vi "SelectRobotConfig.vi"(1 "RobotID":T19) -> (0 "RobotConfig":T1={"Motors"={"RightDrivePrimary"={"CAN Address"=0, "Invert"=FALSE, "InvertSensor"=FALSE, "Unit Conversion Factor"=0.0, "Brake Mode"=enum."Override to Brake", "Reverse Limt Switch Mode"=enum."Disabled", "Forward Limt Swith Mode"=enum."Disabled", "PWM Channel"=enum."Invalid", "Motor Controller Type"=enum."Talon SRX", "Peak Current (A)"=0, "Continuous Current (A)"=0, "Peak Duration (ms)"=0, "Current Limit Enable"=FALSE}, "RightDriveSecondary"={"CAN Address"=0, "Invert"=FALSE, "InvertSensor"=FALSE, "Unit Conversion Factor"=0.0, "Brake Mode"=enum."Override to Brake", "Reverse Limt Switch Mode"=enum."Disabled", "Forward Limt Swith Mode"=enum."Disabled", "PWM Channel"=enum."Invalid", "Motor Controller Type"=enum."Talon SRX", "Peak Current (A)"=0, "Continuous Current (A)"=0, "Peak Duration (ms)"=0, "Current Limit Enable"=FALSE}, "LeftDrivePrimary"={"CAN Address"=0, "Invert"=FALSE, "InvertSensor"=FALSE, "Unit Conversion Factor"=0.0, "Brake Mode"=enum."Override to Brake", "Reverse Limt Switch Mode"=enum."Disabled", "Forward Limt Swith Mode"=enum."Disabled", "PWM Channel"=enum."Invalid", "Motor Controller Type"=enum."Talon SRX", "Peak Current (A)"=0, "Continuous Current (A)"=0, "Peak Duration (ms)"=0, "Current Limit Enable"=FALSE}, "LeftDriveSecondary"={"CAN Address"=0, "Invert"=FALSE, "InvertSensor"=FALSE, "Unit Conversion Factor"=0.0, "Brake Mode"=enum."Override to Brake", "Reverse Limt Switch Mode"=enum."Disabled", "Forward Limt Swith Mode"=enum."Disabled", "PWM Channel"=enum."Invalid", "Motor Controller Type"=enum."Talon SRX", "Peak Current (A)"=0, "Continuous Current (A)"=0, "Peak Duration (ms)"=0, "Current Limit Enable"=FALSE}, "RightShooter"={"CAN Address"=0, "Invert"=FALSE, "InvertSensor"=FALSE, "Unit Conversion Factor"=0.0, "Brake Mode"=enum."Override to Brake", "Reverse Limt Switch Mode"=enum."Disabled", "Forward Limt Swith Mode"=enum."Disabled", "PWM Channel"=enum."Invalid", "Motor Controller Type"=enum."Talon SRX", "Peak Current (A)"=0, "Continuous Current (A)"=0, "Peak Duration (ms)"=0, "Current Limit Enable"=FALSE}, "LeftShooter"={"CAN Address"=0, "Invert"=FALSE, "InvertSensor"=FALSE, "Unit Conversion Factor"=0.0, "Brake Mode"=enum."Override to Brake", "Reverse Limt Switch Mode"=enum."Disabled", "Forward Limt Swith Mode"=enum."Disabled", "PWM Channel"=enum."Invalid", "Motor Controller Type"=enum."Talon SRX", "Peak Current (A)"=0, "Continuous Current (A)"=0, "Peak Duration (ms)"=0, "Current Limit Enable"=FALSE}, "ShooterRotate"={"CAN Address"=0, "Invert"=FALSE, "InvertSensor"=FALSE, "Unit Conversion Factor"=0.0, "Brake Mode"=enum."Override to Brake", "Reverse Limt Switch Mode"=enum."Disabled", "Forward Limt Swith Mode"=enum."Disabled", "PWM Channel"=enum."Invalid", "Motor Controller Type"=enum."Talon SRX", "Peak Current (A)"=0, "Continuous Current (A)"=0, "Peak Duration (ms)"=0, "Current Limit Enable"=FALSE}, "ShooterHood"={"CAN Address"=0, "Invert"=FALSE, "InvertSensor"=FALSE, "Unit Conversion Factor"=0.0, "Brake Mode"=enum."Override to Brake", "Reverse Limt Switch Mode"=enum."Disabled", "Forward Limt Swith Mode"=enum."Disabled", "PWM Channel"=enum."Invalid", "Motor Controller Type"=enum."Talon SRX", "Peak Current (A)"=0, "Continuous Current (A)"=0, "Peak Duration (ms)"=0, "Current Limit Enable"=FALSE}, "HopperWheel"={"CAN Address"=0, "Invert"=FALSE, "InvertSensor"=FALSE, "Unit Conversion Factor"=0.0, "Brake Mode"=enum."Override to Brake", "Reverse Limt Switch Mode"=enum."Disabled", "Forward Limt Swith Mode"=enum."Disabled", "PWM Channel"=enum."Invalid", "Motor Controller Type"=enum."Talon SRX", "Peak Current (A)"=0, "Continuous Current (A)"=0, "Peak Duration (ms)"=0, "Current Limit Enable"=FALSE}, "Elevator"={"CAN Address"=0, "Invert"=FALSE, "InvertSensor"=FALSE, "Unit Conversion Factor"=0.0, "Brake Mode"=enum."Override to Brake", "Reverse Limt Switch Mode"=enum."Disabled", "Forward Limt Swith Mode"=enum."Disabled", "PWM Channel"=enum."Invalid", "Motor Controller Type"=enum."Talon SRX", "Peak Current (A)"=0, "Continuous Current (A)"=0, "Peak Duration (ms)"=0, "Current Limit Enable"=FALSE}, "ClimberLeft"={"CAN Address"=0, "Invert"=FALSE, "InvertSensor"=FALSE, "Unit Conversion Factor"=0.0, "Brake Mode"=enum."Override to Brake", "Reverse Limt Switch Mode"=enum."Disabled", "Forward Limt Swith Mode"=enum."Disabled", "PWM Channel"=enum."Invalid", "Motor Controller Type"=enum."Talon SRX", "Peak Current (A)"=0, "Continuous Current (A)"=0, "Peak Duration (ms)"=0, "Current Limit Enable"=FALSE}, "ClimberRight"={"CAN Address"=0, "Invert"=FALSE, "InvertSensor"=FALSE, "Unit Conversion Factor"=0.0, "Brake Mode"=enum."Override to Brake", "Reverse Limt Switch Mode"=enum."Disabled", "Forward Limt Swith Mode"=enum."Disabled", "PWM Channel"=enum."Invalid", "Motor Controller Type"=enum."Talon SRX", "Peak Current (A)"=0, "Continuous Current (A)"=0, "Peak Duration (ms)"=0, "Current Limit Enable"=FALSE}, "Intake"={"CAN Address"=0, "Invert"=FALSE, "InvertSensor"=FALSE, "Unit Conversion Factor"=0.0, "Brake Mode"=enum."Override to Brake", "Reverse Limt Switch Mode"=enum."Disabled", "Forward Limt Swith Mode"=enum."Disabled", "PWM Channel"=enum."Invalid", "Motor Controller Type"=enum."Talon SRX", "Peak Current (A)"=0, "Continuous Current (A)"=0, "Peak Duration (ms)"=0, "Current Limit Enable"=FALSE}, "ControlPanel"={"CAN Address"=0, "Invert"=FALSE, "InvertSensor"=FALSE, "Unit Conversion Factor"=0.0, "Brake Mode"=enum."Override to Brake", "Reverse Limt Switch Mode"=enum."Disabled", "Forward Limt Swith Mode"=enum."Disabled", "PWM Channel"=enum."Invalid", "Motor Controller Type"=enum."Talon SRX", "Peak Current (A)"=0, "Continuous Current (A)"=0, "Peak Duration (ms)"=0, "Current Limit Enable"=FALSE}}, "PID"={"Shooter"={"P"=0.0, "I"=0.0, "D"=0.0, "F"=0.0, "IZone"=0.0}, "Turret"={"P"=0.0, "I"=0.0, "D"=0.0, "F"=0.0, "IZone"=0.0}, "Elevator"={"P"=0.0, "I"=0.0, "D"=0.0, "F"=0.0, "IZone"=0.0}, "ControlPanel"={"P"=0.0, "I"=0.0, "D"=0.0, "F"=0.0, "IZone"=0.0}, "Hood"={"P"=0.0, "I"=0.0, "D"=0.0, "F"=0.0, "IZone"=0.0}}, "MotionMagic"={"Turret"={"CruiseVelocity"=0, "Acceleration"=0}, "Elevator"={"CruiseVelocity"=0, "Acceleration"=0}, "ControlPanel"={"CruiseVelocity"=0, "Acceleration"=0}}, "Sensors"={"IMU"={"Yaw Axis"=enum."Z", "SPI Bus"=enum."SPI MXP", "AHRS Algorithm"=enum."Complementary", "Calibration Time (s)"=3.0, "Calibrate On Open"=TRUE}, "ElevatorBottom"={"ID"=0, "RangingMode"=enum."Short", "sampleTime(ms)"=24.0}, "ElevatorTop"={"ID"=0, "RangingMode"=enum."Short", "sampleTime(ms)"=24.0}, "ControlPanelColorSensor"={"alsIntegrationTime(ms)"=10.0, "alsGain"=40, "I2C Bus"=enum."I2C On-Board", "numProximityPulses"=5, "proximityGain"=1, "proximityLEDCurrent(mA)"=50, "proximityPulseLength(ms)"=0.01, "proximitySampleTime(ms)"=10.0}}, "Solenoids"={"Intake"={"SolenoidChannel"=enum."Solenoid 0", "Invert"=FALSE}, "ClimberRachet"={"SolenoidChannel"=enum."Solenoid 0", "Invert"=FALSE}}, "EnableCompressor"=FALSE, "RobotDimensions"={"Wheelbase(in)"=0.0, "Length(in)"=0.0}, "CameraMounting"={"LensHeight(in)"=0.0, "RotationRadius(in)"=0.0, "Pitch(deg)"=0.0}, "SensorCalibrations"={"TopToFMinBallDistance(in)"=0.0, "BottomToFMinBallDistance(in)"=0.0}, "Homing"={"Hood Homing Position (deg)"=0.0, "Turret Homing Position (deg)"=0.0}, "MotionLimits"={"Hood"={"Min (deg)"=0.0, "Max (deg)"=0.0}, "Turret"={"Min (deg)"=0.0, "Max (deg)"=0.0}}} {"Sensors"."ElevatorTop"."sampleTime(ms)" min=24.0 max=1000.0 step=1.0; "Sensors"."ElevatorBottom"."sampleTime(ms)" min=24.0 max=1000.0 step=1.0})   [LabVIEW 2019]
uses:
  TypeDefs/RobotID.ctl
  TypeDefs/ConfigComponents/Config_Robot.ctl
  ArgosLib/Config/ConfigComponents/TypeDefs/Config_Motor.ctl
  <vilib>/Rock Robotics/WPI/ThirdParty/Phoenix-LabVIEW/Motor Controller/Controls/CTRE_Phoenix_MotorControl_NeutralMode.ctl
  <vilib>/Rock Robotics/WPI/ThirdParty/Phoenix-LabVIEW/Motor Controller/Controls/CTRE_Phoenix_MotorControl_LimitSwitchNormal.ctl
  <vilib>/Rock Robotics/SystemInterfaces/DIO/FPGA_DIOPWMChannel.ctl
  ArgosLib/Config/ConfigComponents/TypeDefs/Config_MotorCtrlType.ctl
  ArgosLib/Config/ConfigComponents/TypeDefs/Config_PIDParams.ctl
  ArgosLib/Config/ConfigComponents/TypeDefs/Config_MotionMagicParams.ctl
  ArgosLib/Config/ConfigComponents/TypeDefs/Config_IMU.ctl
  <vilib>/Rock Robotics/SystemInterfaces/spilib/spi_bus.ctl
  ArgosLib/Config/ConfigComponents/TypeDefs/Config_PwFToF.ctl
  <vilib>/Playing With Fusion Inc/Playing With Fusion Lib for FRC/PWF_ToF_LabVIEW/Public/TypeDefs/PwF_ToF_RangingMode.ctl
  ArgosLib/Config/ConfigComponents/TypeDefs/Config_PwF_TMD37003.ctl
  <vilib>/Rock Robotics/SystemInterfaces/i2clib/i2c_bus.ctl
  ArgosLib/Config/ConfigComponents/TypeDefs/Config_SingleSolenoid.ctl
  <vilib>/Rock Robotics/WPI/Solenoid/WPI_SolenoidChannel.ctl
  TypeDefs/ConfigComponents/Config_RobotDimensions.ctl
  TypeDefs/ConfigComponents/Config_CameraMounting.ctl
  ArgosLib/ArgosLib.lvlib
  <vilib>/Playing With Fusion Inc/Playing With Fusion Lib for FRC/PWF_ToF_LabVIEW/PwF_ToF.lvlib
panel:
  in  "Competition":T1={"Motors"={"RightDrivePrimary"={"CAN Address"=1, "Invert"=TRUE, "InvertSensor"=FALSE, "Unit Conversion Factor"=0.4342, "Brake Mode"=enum."Override to Brake", "Reverse Limt Switch Mode"=enum."Disabled", "Forward Limt Swith Mode"=enum."Disabled", "PWM Channel"=enum."Invalid", "Motor Controller Type"=enum."Venom", "Peak Current (A)"=0, "Continuous Current (A)"=0, "Peak Duration (ms)"=0, "Current Limit Enable"=FALSE}, "RightDriveSecondary"={"CAN Address"=2, "Invert"=TRUE, "InvertSensor"=FALSE, "Unit Conversion Factor"=0.4342, "Brake Mode"=enum."Override to Brake", "Reverse Limt Switch Mode"=enum."Disabled", "Forward Limt Swith Mode"=enum."Disabled", "PWM Channel"=enum."Invalid", "Motor Controller Type"=enum."Venom", "Peak Current (A)"=0, "Continuous Current (A)"=0, "Peak Duration (ms)"=0, "Current Limit Enable"=FALSE}, "LeftDrivePrimary"={"CAN Address"=3, "Invert"=FALSE, "InvertSensor"=FALSE, "Unit Conversion Factor"=0.4342, "Brake Mode"=enum."Override to Brake", "Reverse Limt Switch Mode"=enum."Disabled", "Forward Limt Swith Mode"=enum."Disabled", "PWM Channel"=enum."Invalid", "Motor Controller Type"=enum."Venom", "Peak Current (A)"=0, "Continuous Current (A)"=0, "Peak Duration (ms)"=0, "Current Limit Enable"=FALSE}, "LeftDriveSecondary"={"CAN Address"=4, "Invert"=FALSE, "InvertSensor"=FALSE, "Unit Conversion Factor"=0.4342, "Brake Mode"=enum."Override to Brake", "Reverse Limt Switch Mode"=enum."Disabled", "Forward Limt Swith Mode"=enum."Disabled", "PWM Channel"=enum."Invalid", "Motor Controller Type"=enum."Venom", "Peak Current (A)"=0, "Continuous Current (A)"=0, "Peak Duration (ms)"=0, "Current Limit Enable"=FALSE}, "RightShooter"={"CAN Address"=5, "Invert"=FALSE, "InvertSensor"=FALSE, "Unit Conversion Factor"=1228.8, "Brake Mode"=enum."Override to Coast", "Reverse Limt Switch Mode"=enum."Disabled", "Forward Limt Swith Mode"=enum."Disabled", "PWM Channel"=enum."Invalid", "Motor Controller Type"=enum."Falcon FX", "Peak Current (A)"=0, "Continuous Current (A)"=0, "Peak Duration (ms)"=0, "Current Limit Enable"=FALSE}, "LeftShooter"={"CAN Address"=6, "Invert"=TRUE, "InvertSensor"=FALSE, "Unit Conversion Factor"=1228.8, "Brake Mode"=enum."Override to Coast", "Reverse Limt Switch Mode"=enum."Disabled", "Forward Limt Swith Mode"=enum."Disabled", "PWM Channel"=enum."Invalid", "Motor Controller Type"=enum."Falcon FX", "Peak Current (A)"=0, "Continuous Current (A)"=0, "Peak Duration (ms)"=0, "Current Limit Enable"=FALSE}, "ShooterRotate"={"CAN Address"=7, "Invert"=TRUE, "InvertSensor"=TRUE, "Unit Conversion Factor"=11.3777, "Brake Mode"=enum."Override to Brake", "Reverse Limt Switch Mode"=enum."Disabled", "Forward Limt Swith Mode"=enum."Disabled", "PWM Channel"=enum."Invalid", "Motor Controller Type"=enum."Talon SRX", "Peak Current (A)"=0, "Continuous Current (A)"=0, "Peak Duration (ms)"=0, "Current Limit Enable"=FALSE}, "ShooterHood"={"CAN Address"=8, "Invert"=FALSE, "InvertSensor"=FALSE, "Unit Conversion Factor"=153.949, "Brake Mode"=enum."Override to Brake", "Reverse Limt Switch Mode"=enum."Disabled", "Forward Limt Swith Mode"=enum."Disabled", "PWM Channel"=enum."Invalid", "Motor Controller Type"=enum."Talon SRX", "Peak Current (A)"=0, "Continuous Current (A)"=0, "Peak Duration (ms)"=0, "Current Limit Enable"=FALSE}, "HopperWheel"={"CAN Address"=9, "Invert"=FALSE, "InvertSensor"=FALSE, "Unit Conversion Factor"=0.0, "Brake Mode"=enum."Override to Brake", "Reverse Limt Switch Mode"=enum."Disabled", "Forward Limt Swith Mode"=enum."Disabled", "PWM Channel"=enum."Invalid", "Motor Controller Type"=enum."Talon SRX", "Peak Current (A)"=0, "Continuous Current (A)"=0, "Peak Duration (ms)"=0, "Current Limit Enable"=FALSE}, "Elevator"={"CAN Address"=10, "Invert"=FALSE, "InvertSensor"=FALSE, "Unit Conversion Factor"=0.0, "Brake Mode"=enum."Override to Brake", "Reverse Limt Switch Mode"=enum."Disabled", "Forward Limt Swith Mode"=enum."Disabled", "PWM Channel"=enum."Invalid", "Motor Controller Type"=enum."Talon SRX", "Peak Current (A)"=0, "Continuous Current (A)"=0, "Peak Duration (ms)"=0, "Current Limit Enable"=FALSE}, "ClimberLeft"={"CAN Address"=11, "Invert"=TRUE, "InvertSensor"=FALSE, "Unit Conversion Factor"=0.0, "Brake Mode"=enum."Override to Brake", "Reverse Limt Switch Mode"=enum."Disabled", "Forward Limt Swith Mode"=enum."Disabled", "PWM Channel"=enum."Invalid", "Motor Controller Type"=enum."Talon SRX", "Peak Current (A)"=0, "Continuous Current (A)"=0, "Peak Duration (ms)"=0, "Current Limit Enable"=FALSE}, "ClimberRight"={"CAN Address"=12, "Invert"=FALSE, "InvertSensor"=FALSE, "Unit Conversion Factor"=0.0, "Brake Mode"=enum."Override to Brake", "Reverse Limt Switch Mode"=enum."Disabled", "Forward Limt Swith Mode"=enum."Disabled", "PWM Channel"=enum."Invalid", "Motor Controller Type"=enum."Talon SRX", "Peak Current (A)"=0, "Continuous Current (A)"=0, "Peak Duration (ms)"=0, "Current Limit Enable"=FALSE}, "Intake"={"CAN Address"=13, "Invert"=TRUE, "InvertSensor"=FALSE, "Unit Conversion Factor"=0.0, "Brake Mode"=enum."Override to Brake", "Reverse Limt Switch Mode"=enum."Disabled", "Forward Limt Swith Mode"=enum."Disabled", "PWM Channel"=enum."Invalid", "Motor Controller Type"=enum."Talon SRX", "Peak Current (A)"=0, "Continuous Current (A)"=0, "Peak Duration (ms)"=0, "Current Limit Enable"=FALSE}, "ControlPanel"={"CAN Address"=14, "Invert"=FALSE, "InvertSensor"=FALSE, "Unit Conversion Factor"=0.0, "Brake Mode"=enum."Override to Brake", "Reverse Limt Switch Mode"=enum."Disabled", "Forward Limt Swith Mode"=enum."Disabled", "PWM Channel"=enum."Invalid", "Motor Controller Type"=enum."Talon SRX", "Peak Current (A)"=0, "Continuous Current (A)"=0, "Peak Duration (ms)"=0, "Current Limit Enable"=FALSE}}, "PID"={"Shooter"={"P"=1.0, "I"=0.001, "D"=0.0, "F"=0.055, "IZone"=200.0}, "Turret"={"P"=6.0, "I"=0.1, "D"=0.0, "F"=0.0, "IZone"=500.0}, "Elevator"={"P"=0.0, "I"=0.0, "D"=0.0, "F"=0.0, "IZone"=0.0}, "ControlPanel"={"P"=0.0, "I"=0.0, "D"=0.0, "F"=0.0, "IZone"=0.0}, "Hood"={"P"=0.5, "I"=0.0007, "D"=0.0, "F"=0.0, "IZone"=200.0}}, "MotionMagic"={"Turret"={"CruiseVelocity"=0, "Acceleration"=0}, "Elevator"={"CruiseVelocity"=0, "Acceleration"=0}, "ControlPanel"={"CruiseVelocity"=0, "Acceleration"=0}}, "Sensors"={"IMU"={"Yaw Axis"=enum."Z", "SPI Bus"=enum."SPI MXP", "AHRS Algorithm"=enum."Complementary", "Calibration Time (s)"=3.0, "Calibrate On Open"=TRUE}, "ElevatorBottom"={"ID"=1, "RangingMode"=enum."Short", "sampleTime(ms)"=24.0}, "ElevatorTop"={"ID"=2, "RangingMode"=enum."Short", "sampleTime(ms)"=24.0}, "ControlPanelColorSensor"={"alsIntegrationTime(ms)"=10.0, "alsGain"=40, "I2C Bus"=enum."I2C On-Board", "numProximityPulses"=5, "proximityGain"=1, "proximityLEDCurrent(mA)"=50, "proximityPulseLength(ms)"=0.01, "proximitySampleTime(ms)"=10.0}}, "Solenoids"={"Intake"={"SolenoidChannel"=enum."Solenoid 0", "Invert"=FALSE}, "ClimberRachet"={"SolenoidChannel"=enum."Solenoid 1", "Invert"=FALSE}}, "EnableCompressor"=TRUE, "RobotDimensions"={"Wheelbase(in)"=0.0, "Length(in)"=0.0}, "CameraMounting"={"LensHeight(in)"=37.75, "RotationRadius(in)"=7.0, "Pitch(deg)"=24.5}, "SensorCalibrations"={"TopToFMinBallDistance(in)"=1.0, "BottomToFMinBallDistance(in)"=0.0}, "Homing"={"Hood Homing Position (deg)"=45.0, "Turret Homing Position (deg)"=0.0}, "MotionLimits"={"Hood"={"Min (deg)"=47.0, "Max (deg)"=72.0}, "Turret"={"Min (deg)"=-108.0, "Max (deg)"=108.0}}} {"Sensors"."ElevatorTop"."sampleTime(ms)" min=24.0 max=1000.0 step=1.0; "Sensors"."ElevatorBottom"."sampleTime(ms)" min=24.0 max=1000.0 step=1.0}
  in  "Practice":T1={"Motors"={"RightDrivePrimary"={"CAN Address"=1, "Invert"=TRUE, "InvertSensor"=FALSE, "Unit Conversion Factor"=0.4342, "Brake Mode"=enum."Override to Brake", "Reverse Limt Switch Mode"=enum."Disabled", "Forward Limt Swith Mode"=enum."Disabled", "PWM Channel"=enum."Invalid", "Motor Controller Type"=enum."Venom", "Peak Current (A)"=0, "Continuous Current (A)"=0, "Peak Duration (ms)"=0, "Current Limit Enable"=FALSE}, "RightDriveSecondary"={"CAN Address"=2, "Invert"=TRUE, "InvertSensor"=FALSE, "Unit Conversion Factor"=0.4342, "Brake Mode"=enum."Override to Brake", "Reverse Limt Switch Mode"=enum."Disabled", "Forward Limt Swith Mode"=enum."Disabled", "PWM Channel"=enum."Invalid", "Motor Controller Type"=enum."Venom", "Peak Current (A)"=0, "Continuous Current (A)"=0, "Peak Duration (ms)"=0, "Current Limit Enable"=FALSE}, "LeftDrivePrimary"={"CAN Address"=3, "Invert"=FALSE, "InvertSensor"=FALSE, "Unit Conversion Factor"=0.4342, "Brake Mode"=enum."Override to Brake", "Reverse Limt Switch Mode"=enum."Disabled", "Forward Limt Swith Mode"=enum."Disabled", "PWM Channel"=enum."Invalid", "Motor Controller Type"=enum."Venom", "Peak Current (A)"=0, "Continuous Current (A)"=0, "Peak Duration (ms)"=0, "Current Limit Enable"=FALSE}, "LeftDriveSecondary"={"CAN Address"=4, "Invert"=FALSE, "InvertSensor"=FALSE, "Unit Conversion Factor"=0.4342, "Brake Mode"=enum."Override to Brake", "Reverse Limt Switch Mode"=enum."Disabled", "Forward Limt Swith Mode"=enum."Disabled", "PWM Channel"=enum."Invalid", "Motor Controller Type"=enum."Venom", "Peak Current (A)"=0, "Continuous Current (A)"=0, "Peak Duration (ms)"=0, "Current Limit Enable"=FALSE}, "RightShooter"={"CAN Address"=5, "Invert"=TRUE, "InvertSensor"=FALSE, "Unit Conversion Factor"=1228.8, "Brake Mode"=enum."Override to Coast", "Reverse Limt Switch Mode"=enum."Disabled", "Forward Limt Swith Mode"=enum."Disabled", "PWM Channel"=enum."Invalid", "Motor Controller Type"=enum."Falcon FX", "Peak Current (A)"=0, "Continuous Current (A)"=0, "Peak Duration (ms)"=0, "Current Limit Enable"=FALSE}, "LeftShooter"={"CAN Address"=6, "Invert"=FALSE, "InvertSensor"=FALSE, "Unit Conversion Factor"=1228.8, "Brake Mode"=enum."Override to Coast", "Reverse Limt Switch Mode"=enum."Disabled", "Forward Limt Swith Mode"=enum."Disabled", "PWM Channel"=enum."Invalid", "Motor Controller Type"=enum."Falcon FX", "Peak Current (A)"=0, "Continuous Current (A)"=0, "Peak Duration (ms)"=0, "Current Limit Enable"=FALSE}, "ShooterRotate"={"CAN Address"=7, "Invert"=TRUE, "InvertSensor"=FALSE, "Unit Conversion Factor"=11.3777, "Brake Mode"=enum."Override to Brake", "Reverse Limt Switch Mode"=enum."Disabled", "Forward Limt Swith Mode"=enum."Disabled", "PWM Channel"=enum."Invalid", "Motor Controller Type"=enum."Talon SRX", "Peak Current (A)"=0, "Continuous Current (A)"=0, "Peak Duration (ms)"=0, "Current Limit Enable"=FALSE}, "ShooterHood"={"CAN Address"=8, "Invert"=FALSE, "InvertSensor"=FALSE, "Unit Conversion Factor"=442.112, "Brake Mode"=enum."Override to Brake", "Reverse Limt Switch Mode"=enum."Disabled", "Forward Limt Swith Mode"=enum."Disabled", "PWM Channel"=enum."Invalid", "Motor Controller Type"=enum."Talon SRX", "Peak Current (A)"=0, "Continuous Current (A)"=0, "Peak Duration (ms)"=0, "Current Limit Enable"=FALSE}, "HopperWheel"={"CAN Address"=9, "Invert"=FALSE, "InvertSensor"=FALSE, "Unit Conversion Factor"=0.0, "Brake Mode"=enum."Override to Brake", "Reverse Limt Switch Mode"=enum."Disabled", "Forward Limt Swith Mode"=enum."Disabled", "PWM Channel"=enum."Invalid", "Motor Controller Type"=enum."Talon SRX", "Peak Current (A)"=0, "Continuous Current (A)"=0, "Peak Duration (ms)"=0, "Current Limit Enable"=FALSE}, "Elevator"={"CAN Address"=10, "Invert"=FALSE, "InvertSensor"=FALSE, "Unit Conversion Factor"=0.0, "Brake Mode"=enum."Override to Brake", "Reverse Limt Switch Mode"=enum."Disabled", "Forward Limt Swith Mode"=enum."Disabled", "PWM Channel"=enum."Invalid", "Motor Controller Type"=enum."Talon SRX", "Peak Current (A)"=0, "Continuous Current (A)"=0, "Peak Duration (ms)"=0, "Current Limit Enable"=FALSE}, "ClimberLeft"={"CAN Address"=11, "Invert"=FALSE, "InvertSensor"=FALSE, "Unit Conversion Factor"=0.0, "Brake Mode"=enum."Override to Brake", "Reverse Limt Switch Mode"=enum."Disabled", "Forward Limt Swith Mode"=enum."Disabled", "PWM Channel"=enum."Invalid", "Motor Controller Type"=enum."Talon SRX", "Peak Current (A)"=0, "Continuous Current (A)"=0, "Peak Duration (ms)"=0, "Current Limit Enable"=FALSE}, "ClimberRight"={"CAN Address"=12, "Invert"=FALSE, "InvertSensor"=FALSE, "Unit Conversion Factor"=0.0, "Brake Mode"=enum."Override to Brake", "Reverse Limt Switch Mode"=enum."Disabled", "Forward Limt Swith Mode"=enum."Disabled", "PWM Channel"=enum."Invalid", "Motor Controller Type"=enum."Talon SRX", "Peak Current (A)"=0, "Continuous Current (A)"=0, "Peak Duration (ms)"=0, "Current Limit Enable"=FALSE}, "Intake"={"CAN Address"=13, "Invert"=TRUE, "InvertSensor"=FALSE, "Unit Conversion Factor"=0.0, "Brake Mode"=enum."Override to Brake", "Reverse Limt Switch Mode"=enum."Disabled", "Forward Limt Swith Mode"=enum."Disabled", "PWM Channel"=enum."Invalid", "Motor Controller Type"=enum."Talon SRX", "Peak Current (A)"=0, "Continuous Current (A)"=0, "Peak Duration (ms)"=0, "Current Limit Enable"=FALSE}, "ControlPanel"={"CAN Address"=14, "Invert"=FALSE, "InvertSensor"=FALSE, "Unit Conversion Factor"=0.0, "Brake Mode"=enum."Override to Brake", "Reverse Limt Switch Mode"=enum."Disabled", "Forward Limt Swith Mode"=enum."Disabled", "PWM Channel"=enum."Invalid", "Motor Controller Type"=enum."Talon SRX", "Peak Current (A)"=0, "Continuous Current (A)"=0, "Peak Duration (ms)"=0, "Current Limit Enable"=FALSE}}, "PID"={"Shooter"={"P"=0.0004, "I"=1e-06, "D"=0.0, "F"=0.0002, "IZone"=200.0}, "Turret"={"P"=6.0, "I"=0.007, "D"=0.0, "F"=0.0, "IZone"=500.0}, "Elevator"={"P"=0.0, "I"=0.0, "D"=0.0, "F"=0.0, "IZone"=0.0}, "ControlPanel"={"P"=0.0, "I"=0.0, "D"=0.0, "F"=0.0, "IZone"=0.0}, "Hood"={"P"=0.3, "I"=0.0001, "D"=0.0, "F"=0.0, "IZone"=1000.0}}, "MotionMagic"={"Turret"={"CruiseVelocity"=0, "Acceleration"=0}, "Elevator"={"CruiseVelocity"=0, "Acceleration"=0}, "ControlPanel"={"CruiseVelocity"=0, "Acceleration"=0}}, "Sensors"={"IMU"={"Yaw Axis"=enum."Z", "SPI Bus"=enum."SPI MXP", "AHRS Algorithm"=enum."Complementary", "Calibration Time (s)"=3.0, "Calibrate On Open"=TRUE}, "ElevatorBottom"={"ID"=1, "RangingMode"=enum."Short", "sampleTime(ms)"=24.0}, "ElevatorTop"={"ID"=2, "RangingMode"=enum."Short", "sampleTime(ms)"=24.0}, "ControlPanelColorSensor"={"alsIntegrationTime(ms)"=10.0, "alsGain"=40, "I2C Bus"=enum."I2C On-Board", "numProximityPulses"=5, "proximityGain"=1, "proximityLEDCurrent(mA)"=50, "proximityPulseLength(ms)"=0.01, "proximitySampleTime(ms)"=10.0}}, "Solenoids"={"Intake"={"SolenoidChannel"=enum."Solenoid 0", "Invert"=TRUE}, "ClimberRachet"={"SolenoidChannel"=enum."Solenoid 1", "Invert"=FALSE}}, "EnableCompressor"=FALSE, "RobotDimensions"={"Wheelbase(in)"=0.0, "Length(in)"=0.0}, "CameraMounting"={"LensHeight(in)"=37.75, "RotationRadius(in)"=7.0, "Pitch(deg)"=22.0}, "SensorCalibrations"={"TopToFMinBallDistance(in)"=1.0, "BottomToFMinBallDistance(in)"=0.0}, "Homing"={"Hood Homing Position (deg)"=44.0, "Turret Homing Position (deg)"=0.0}, "MotionLimits"={"Hood"={"Min (deg)"=47.0, "Max (deg)"=72.0}, "Turret"={"Min (deg)"=-108.0, "Max (deg)"=108.0}}} {"Sensors"."ElevatorTop"."sampleTime(ms)" min=24.0 max=1000.0 step=1.0; "Sensors"."ElevatorBottom"."sampleTime(ms)" min=24.0 max=1000.0 step=1.0}
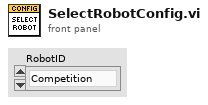
[diagram p1: front panel]
types:
  T1 = typedef "Config_Robot.ctl" = cluster{"Motors":cluster{"RightDrivePrimary":T2, "RightDriveSecondary":T2, "LeftDrivePrimary":T2, "LeftDriveSecondary":T2, "RightShooter":T2, "LeftShooter":T2, "ShooterRotate":T2, "ShooterHood":T2, "HopperWheel":T2, "Elevator":T2, "ClimberLeft":T2, "ClimberRight":T2, "Intake":T2, "ControlPanel":T2}, "PID":cluster{"Shooter":T7, "Turret":T7, "Elevator":T7, "ControlPanel":T7, "Hood":T7}, "MotionMagic":cluster{"Turret":T8, "Elevator":T8, "ControlPanel":T8}, "Sensors":cluster{"IMU":T9, "ElevatorBottom":T11, "ElevatorTop":T11, "ControlPanelColorSensor":T13}, "Solenoids":cluster{"Intake":T15, "ClimberRachet":T15}, "EnableCompressor":bool, "RobotDimensions":T17, "CameraMounting":T18, "SensorCalibrations":cluster{"TopToFMinBallDistance(in)":dbl, "BottomToFMinBallDistance(in)":dbl}, "Homing":cluster{"Hood Homing Position (deg)":dbl, "Turret Homing Position (deg)":dbl}, "MotionLimits":cluster{"Hood":cluster{"Min (deg)":dbl, "Max (deg)":dbl}, "Turret":cluster{"Min (deg)":dbl, "Max (deg)":dbl}}}
  T2 = typedef "ArgosLib.lvlib/Config_Motor.ctl" = cluster{"CAN Address":u8, "Invert":bool, "InvertSensor":bool, "Unit Conversion Factor":dbl, "Brake Mode":T3, "Reverse Limt Switch Mode":T4, "Forward Limt Swith Mode":T4, "PWM Channel":T5, "Motor Controller Type":T6, "Peak Current (A)":i32, "Continuous Current (A)":i32, "Peak Duration (ms)":i32, "Current Limit Enable":bool}
  T3 = typedef "CTRE_Phoenix_MotorControl_NeutralMode.ctl" = enum8{"EEPROMSetting", "Override to Coast", "Override to Brake"}
  T4 = typedef "CTRE_Phoenix_MotorControl_LimitSwitchNormal.ctl" = enum16{"Normally Open", "Normally Closed", "Disabled"}
  T5 = typedef "FPGA_DIOPWMChannel.ctl" = enum8{"PWM 0", "PWM 1", "PWM 2", "PWM 3", "PWM 4", "PWM 5", "PWM 6", "PWM 7", "PWM 8", "PWM 9", "PWM MXP 0", "PWM MXP 1", "PWM MXP 2", "PWM MXP 3", "PWM MXP 4", "PWM MXP 5", "PWM MXP 6", "PWM MXP 7", "PWM MXP 8", "PWM MXP 9", "Invalid"}
  T6 = typedef "ArgosLib.lvlib/Config_MotorCtrlType.ctl" = enum16{"Disabled", "Talon SRX", "Talon SR", "Venom", "Spark MAX", "Falcon FX"}
  T7 = typedef "ArgosLib.lvlib/Config_PIDParams.ctl" = cluster{"P":dbl, "I":dbl, "D":dbl, "F":dbl, "IZone":dbl}
  T8 = typedef "ArgosLib.lvlib/Config_MotionMagicParams.ctl" = cluster{"CruiseVelocity":i32, "Acceleration":i32}
  T9 = typedef "ArgosLib.lvlib/Config_IMU.ctl" = cluster{"Yaw Axis":enum16{"X", "Y", "Z"}, "SPI Bus":T10, "AHRS Algorithm":enum16{"Complementary", "Madgwick"}, "Calibration Time (s)":dbl, "Calibrate On Open":bool}
  T10 = typedef "spi_bus.ctl" = enum16{"SPI On-Board, CS0", "SPI On-Board, CS1", "SPI On-Board, CS2", "SPI On-Board, CS3", "SPI MXP", "Invalid"}
  T11 = typedef "ArgosLib.lvlib/Config_PwFToF.ctl" = cluster{"ID":u8, "RangingMode":T12, "sampleTime(ms)":dbl}
  T12 = typedef "PlayingWithFusionLib.lvlib/PwF_ToF.lvlib/PwF_ToF_RangingMode.ctl" = enum16{"Short", "Medium", "Long"}
  T13 = typedef "ArgosLib.lvlib/Config_PwF_TMD37003.ctl" = cluster{"alsIntegrationTime(ms)":dbl, "alsGain":u8, "I2C Bus":T14, "numProximityPulses":u8, "proximityGain":u8, "proximityLEDCurrent(mA)":u8, "proximityPulseLength(ms)":dbl, "proximitySampleTime(ms)":dbl}
  T14 = typedef "i2c_bus.ctl" = enum16{"I2C On-Board", "I2C MXP", "Invalid"}
  T15 = typedef "ArgosLib.lvlib/Config_SingleSolenoid.ctl" = cluster{"SolenoidChannel":T16, "Invert":bool}
  T16 = typedef "WPI_SolenoidChannel.ctl" = enum8{"Solenoid 0", "Solenoid 1", "Solenoid 2", "Solenoid 3", "Solenoid 4", "Solenoid 5", "Solenoid 6", "Solenoid 7", "Invalid"}
  T17 = typedef "Config_RobotDimensions.ctl" = cluster{"Wheelbase(in)":dbl, "Length(in)":dbl}
  T18 = typedef "Config_CameraMounting.ctl" = cluster{"LensHeight(in)":dbl, "RotationRadius(in)":dbl, "Pitch(deg)":dbl}
  T19 = typedef "RobotID.ctl" = enum16{"Competition", "Practice"}
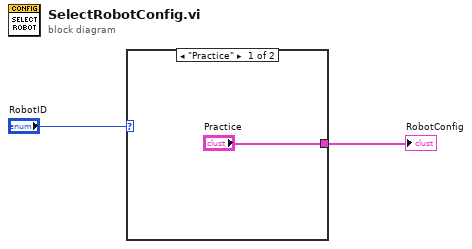
[diagram p0: block diagram]
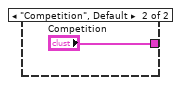
[diagram p2: hidden frame]
diagram:
  n1 = case shown="\"Practice\"" "RobotID" {
    tunnel: ["Practice" "Competition"] -> w1
    frame "Practice" {
    }
    frame "Competition", Default {
    }
  }
  "RobotConfig" <- w1
